vi "Next Step.vi"(8 "error in (no error)":errorcluster, 11 "Voltage Pulse Gating System (HV supply) in":refnum<class "Voltage Pulse Gating System (HV supply).lvclass">) -> (0 "error out":errorcluster, 1 "Current Step":u32, 2 "Current Position":dbl, 3 "Voltage Pulse Gating System (HV supply) out":refnum<class "Voltage Pulse Gating System (HV supply).lvclass">)   [LabVIEW 2023, in "Voltage Pulse Gating System (HV supply).lvclass"]
doc: "(Dynamic) Move to the next preconfigured step of this Scanner, and return the current position (actual, not intended) of this Scanner. Increment the step counter by one."
uses:
  Voltage Pulse Gating System (HV supply).lvclass
  Scanner/Scanner.lvclass
  Instruments/Utility Classes/Scannable/Scannable.lvclass
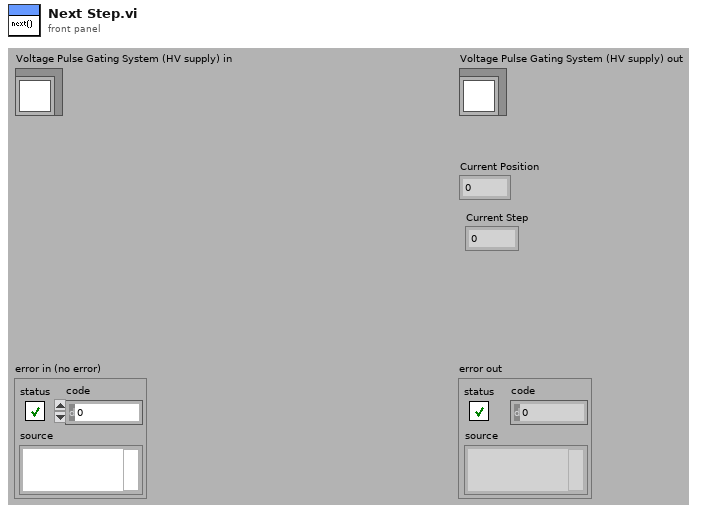
[diagram p1: front panel]
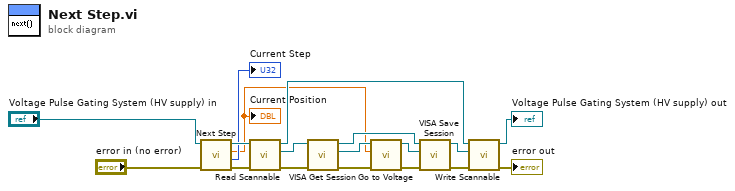
[diagram p0: block diagram]
diagram:
  n1 = call-parent "Next Step.vi"("error in (no error)"="error in (no error)", "Scanner in"="Voltage Pulse Gating System (HV supply) in") -> ("error out"=w12:errorcluster, "Current Step"=→"Current Step":u32, "Current Position"=w1:dbl, "Scanner out"=w18:refnum<class "Voltage Pulse Gating System (HV supply).lvclass">)  [unwired: 6 out]
  "Current Position" <- w1
  n2 = call-dynamic "Read Scannable.vi"("error in (no error)"=w12, "Scanner.lvclass in"=w18) -> ("error out"=w11:errorcluster, "Scannable.lvclass"=w15:refnum<class "Scannable.lvclass">, "Scanner.lvclass out"=w7:refnum<class "Voltage Pulse Gating System (HV supply).lvclass">)  [unwired: 7 out]
  n3 = call-dynamic "VISA Get Session.vi"("error in (no error)"=w11, "Instrument.lvclass in"=w15) -> ("error out"=w3:errorcluster, "VISA Resource Name"=w2:refnum<visa-resource-name>, "Instrument.lvclass out"=w17:refnum<class "Scannable.lvclass">)  [unwired: 7 out]
  n4 = call "Go to Voltage.vi"("error in"=w3, "Set Voltage"=w1, "VISA Resource Name"=w2) -> ("error out"=w4:errorcluster, "VISA resource name out"=w5:refnum<visa-resource-name>)  [unwired: 6 in, 1 out]
  n5 = call-dynamic "VISA Save Session.vi"("error in (no error)"=w4, "VISA Resource Name"=w5, "Instrument.lvclass in"=w17) -> ("error out"=w6:errorcluster, "Instrument.lvclass out"=w16:refnum<class "Scannable.lvclass">)  [unwired: 7 out]
  n6 = call-dynamic "Write Scannable.vi"("error in (no error)"=w6, "Scannable.lvclass"=w16, "Scanner.lvclass in"=w7) -> ("error out"=→"error out":errorcluster, "Scanner.lvclass out"=→"Voltage Pulse Gating System (HV supply) out":refnum<class "Voltage Pulse Gating System (HV supply).lvclass">)  [unwired: 7 out]
